vi "Emballage_chargement_param_produit.vi"(2 "Refnum Ch":refnum<vi>, 5 "entrée d'erreur (pas d'erreur)":errorcluster, 8 "progress":refnum<vi>) -> (16 "Tableau en sortie":string[][](array[string]), 19 "sortie d'erreur":errorcluster)   [LabVIEW 2020]
uses:
  Modules/FS/60_FS_Controles/60_FS_SetGet.ctl
panel:
  out "REMARQUE":string
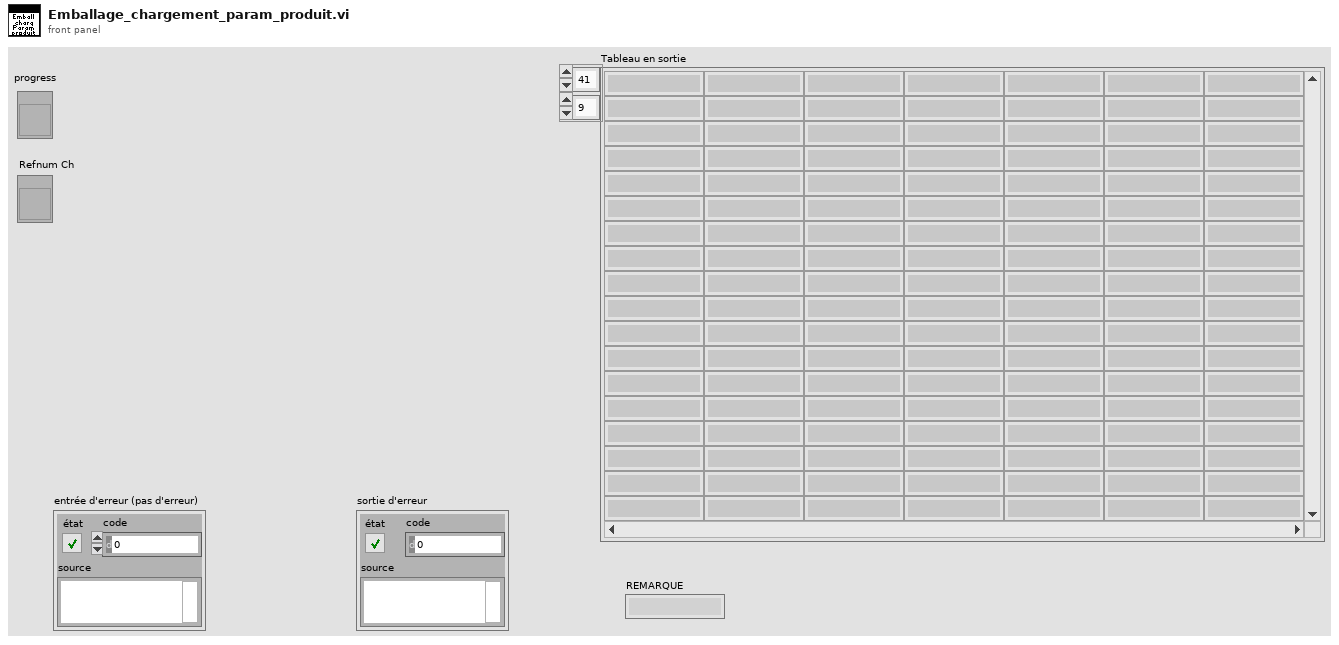
[diagram p1: front panel]
types:
  T1 = typedef "60_FS_SetGet.ctl" = enum16{"set", "get"}
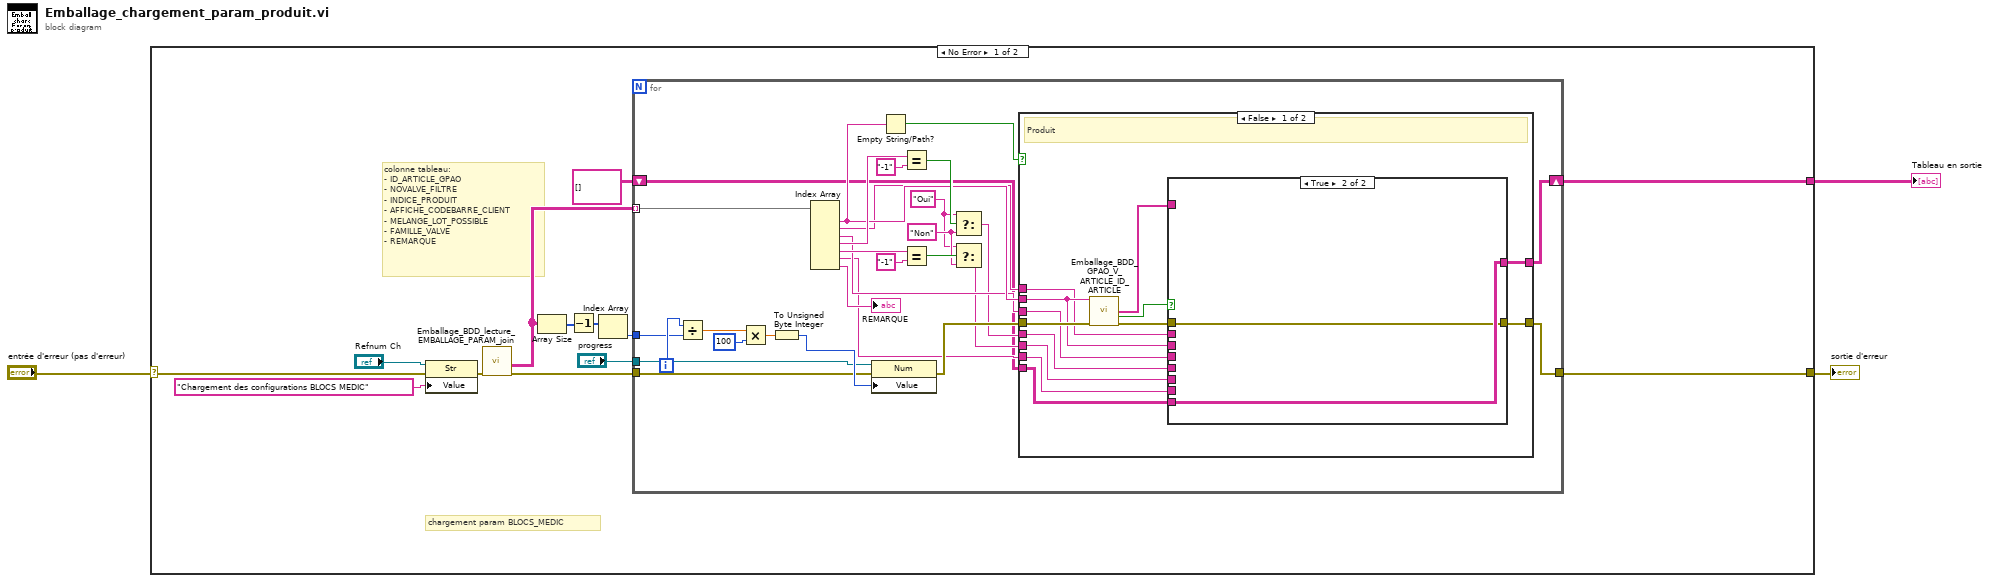
[diagram p0: block diagram]
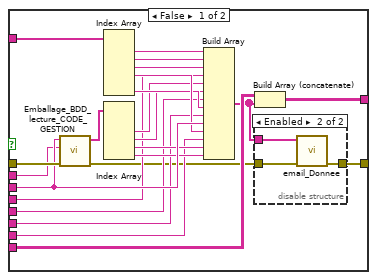
[diagram p2: hidden frame]
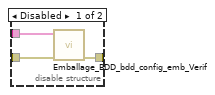
[diagram p3: hidden frame]
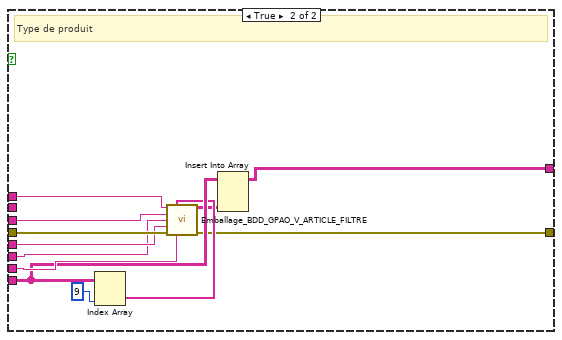
[diagram p4: hidden frame]
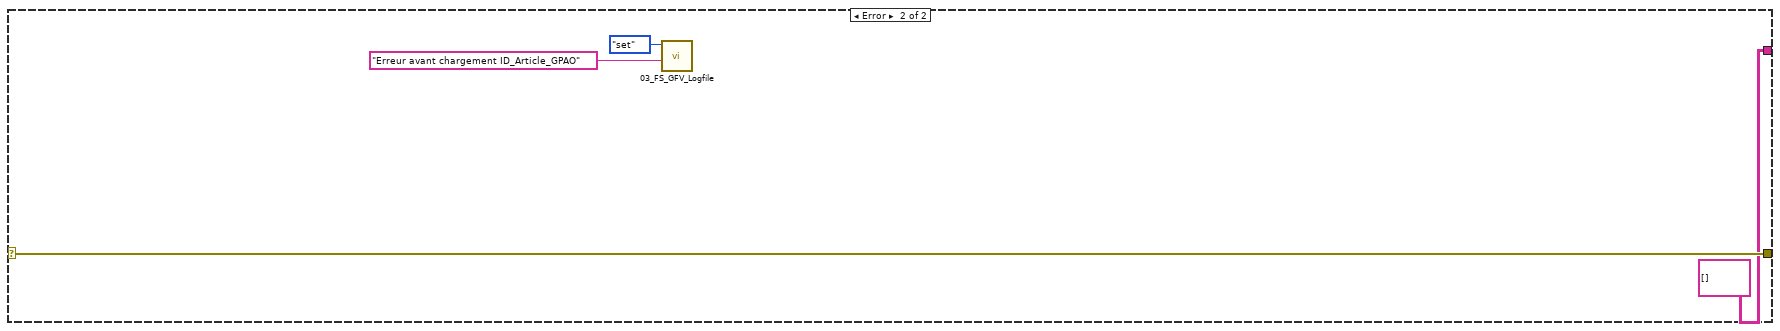
[diagram p5: hidden frame]
diagram:
  n1 = case shown="No Error" "entrée d'erreur (pas d'erreur)" {
    selector: "entrée d'erreur (pas d'erreur)" -> [w15 w105]
    tunnel: [w16 string[][] [] ("Tableau en entrée")] -> w3
    tunnel: [w7 w105] -> w1
    frame No Error {
      # "colonne tableau:\n- ID_ARTICLE_GPAO\n- NOVALVE_FILTRE\n- INDICE_PRODUIT\n- AFFICHE_CODEBARRE_CLIENT\n- MELANGE_LOT_POSSIBLE\n- FAMILLE_VALVE\n- REMARQUE"
      # "chargement param BLOCS_MEDIC"
      n2 = property class="Str"(reference="Refnum Ch", error in=w15, "Value"="Chargement des configurations BLOCS MEDIC" ("Valeur")) -> (error out=w10:errorcluster)  [unwired: 1 out]
      n3 = call "Emballage_BDD_lecture_EMBALLAGE_PARAM_join.vi"("error in"=w10) -> ("error out"=w9:errorcluster, "données"=w8:string[][])  [unwired: 7 in, 2 out]
      n4 = Array Size(array=w8) -> (size(s)=w12:i32[])
      n5 = Decrement(x=w12) -> (x-1=w4:i32[])
      n6 = Index Array(array=w4) -> (element=w11:i32)  [unwired: 1 in]
      n7 = for {
        tunnel: w8 -> [w37] mode=indexing
        tunnel: w9 -> [w39]
        tunnel: w11 -> [w41]
        shift-right: [w17] -> w16
        shift-left: string[][] [] ("Tableau en entrée") -> [w18]
        tunnel: "progress" -> [w38]
        tunnel: [w23] -> w7
        i -> [w42]
        w31 = "Non" ("y")
        w30 = "Oui" ("y")
        n8 = Divide(x=w42, y=w41) -> (x/y=w43:dbl)
        n9 = Multiply(x=w43, y=u8 100) -> (x*y=w45:dbl)
        n10 = To Unsigned Byte Integer(number=w45) -> (unsigned 8bit integer=w40:u8)
        n11 = Index Array(array=w37) -> (element #1=w25:string, element #2=w22:string, element #3=w24:string, element #4=w27:string, element #5=w26:string, element #6=w21:string, element #7=→"REMARQUE":string)  [unwired: 7 in]
        n12 = property class="Num"(reference=w38, error in=w39, "Value"=w40) -> (error out=w34:errorcluster)  [unwired: 1 out]
        n13 = Empty String/Path?(string/path=w25) -> (empty?=w35:bool)
        n14 = Equal?(x=w27, y="-1") -> (x = y?=w32:bool)
        n15 = Equal?(x=w26, y="-1") -> (x = y?=w33:bool)
        n16 = Select(t=w30, s=w32, f=w31) -> (s? t:f=w19:string)
        n17 = Select(t=w30, s=w33, f=w31) -> (s? t:f=w20:string)
        n18 = case shown="False" w35 {
          tunnel: w34 -> [w58 w101]
          tunnel: w25 -> [w55 _]
          tunnel: w24 -> [w54 w99]
          tunnel: [w47 w91] -> w23
          tunnel: w22 -> [w48 w100]
          tunnel: w21 -> [w51 w95]
          tunnel: w20 -> [w52 w96]
          tunnel: w19 -> [w53 w97]
          tunnel: w18 -> [w50 w94]
          tunnel: [w49 w98] -> w17
          frame False {
            # "Produit"
            n19 = call "Emballage_BDD_GPAO_V_ARTICLE_ID_ARTICLE.vi"("ID_ARTICLE"=w55, "error in (no error)"=w58) -> ("Donnée"=w57:string[], "Enr_Annule"=w46:bool, "error out"=w56:errorcluster)  [unwired: 9 in, 2 out]
            n20 = case shown="True" w46 {
              tunnel: w57 -> [w81 _]
              tunnel: w56 -> [w79 w88]
              tunnel: w55 -> [w77 _]
              tunnel: w54 -> [w70 _]
              tunnel: w53 -> [w67 _]
              tunnel: w52 -> [w66 _]
              tunnel: w51 -> [w65 _]
              tunnel: w50 -> [w64 w89]
              tunnel: [w63 w89] -> w49
              tunnel: w48 -> [w62 _]
              tunnel: [w59 w88] -> w47
              frame False {
                n21 = call "Emballage_BDD_lecture_CODE_GESTION.vi"("Error in"=w79, "NOVALVE_FILTRE"=w62, "ID_ARTICLE_GPAO"=w77) -> ("Error out"=w60:errorcluster, "données"=w78:string[])  [unwired: 7 in]
                n22 = Index Array(array=w81) -> (element #1=w80:string, element #2=w68:string, element #3=w69:string, element #4=w74:string, element #6=w73:string)  [unwired: 6 in, 1 out]
                n23 = Index Array(array=w78) -> (element #2=w71:string, element #3=w72:string, element #4=w75:string, element #5=w76:string)  [unwired: 5 in, 1 out]
                n24 = Build Array(w80, w68, w69, w70, w71, w72, w67, w73, w66, w77, w74, w65, w75, w76) -> (w61:string[])
                n25 = Build Array (concatenate)(w64, w61) -> (w63:string[][])
                n26 = disable-structure shown="Enabled" {
                  disable-tunnel: w61 -> [w84 w85]
                  disable-tunnel: w60 -> [w83 w87]
                  disable-tunnel: [w82 w86] -> w59
                  frame Disabled {
                    n27 = call "Emballage_BDD_bdd_config_emb_Verif.vi"("Error in"=w83, "tableau_config"=w84) -> ("Error out"=w82:errorcluster)  [unwired: 9 in]
                  }
                  frame Enabled {
                    n28 = call "email_Donnee.vi"("entrée d'erreur (pas d'erreur)"=w87, "tableau_config"=w85) -> ("sortie d'erreur"=w86:errorcluster)  [unwired: 9 in]
                  }
                }
              }
              frame True {
              }
            }
          }
          frame True {
            # "Type de produit"
            n29 = Index Array(array=w94, index (col)=9 ("index (row)")) -> (element=w92:string[])  [unwired: 1 in]
            n30 = call "Emballage_BDD_GPAO_V_ARTICLE_FILTRE.vi"("NOVALVE_FILTRE"=w100, "tbl_ID_ARTICLE"=w92, "indice_produit"=w99, "Melange_des_lots_possible"=w96, "Affiche_code_barre"=w97, "error in (no error)"=w101, "Famille"=w95) -> ("Donnée Final"=w90:string[][], "error out"=w91:errorcluster)  [unwired: 5 in, 2 out]
            n31 = Insert Into Array(array=w94, new element=w90) -> (w98:string[][])  [unwired: 2 in]
          }
        }
      }
    }
    frame Error {
      n32 = call "03_FS_GFV_Logfile.vi"("Chaîne"="Erreur avant chargement ID_Article_GPAO", "States"=60_FS_SetGet."set") -> ()  [unwired: 8 in, 2 out]
    }
  }
  "Tableau en sortie" <- w3
  "sortie d'erreur" <- w1
